vi "Generate Pulse.vi"(4 "timeout (s)":dbl=10.0 format="%0.2f", 5 "error in":errorcluster, 7 "stop (T)":bool=TRUE, 10 "device name":tag="PXIe-6341") -> (14 "task out":refnum<k21>, 19 "error out":errorcluster)   [LabVIEW 2021]
doc: "Creates, edits, and runs tasks using NI-DAQmx. Refer to the NI-DAQmx Readme for a complete listing of devices NI-DAQmx supports.\n\nWhen you place this Express VI on the block diagram, the DAQ Assistant launches to create a new task. After you create a task, you can double-click the DAQ Assistant Express VI to edit that task. For continuous measurement or generation, place a while loop around the DAQ Assistant Express VI."
uses:
  <vilib>/DAQmx/create/channels.llb/DAQmx Create Channel (CO-Pulse Generation-Time).vi
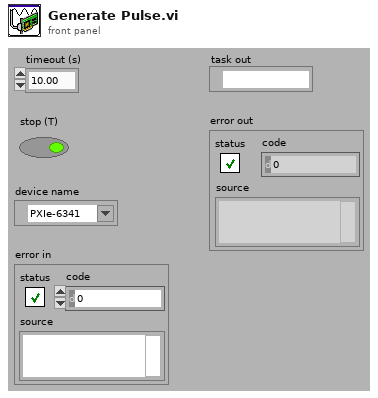
[diagram p1: front panel]
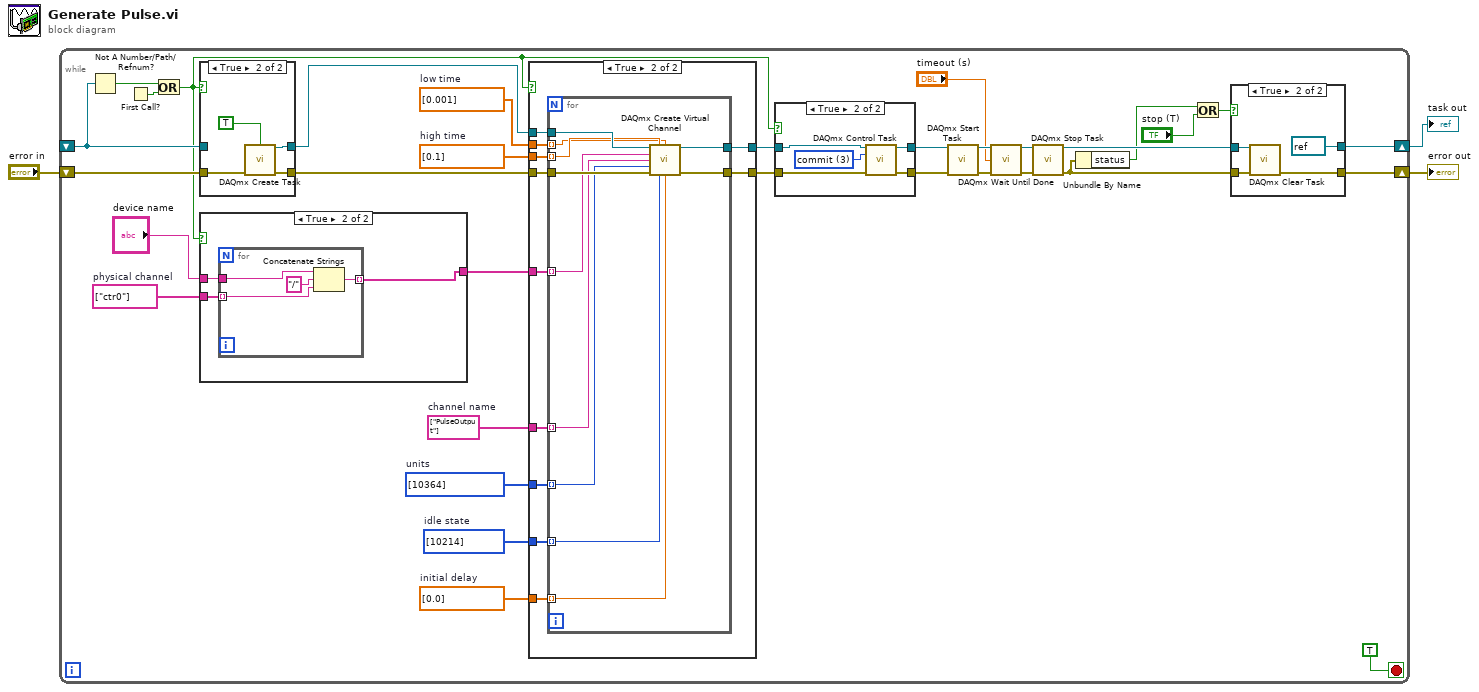
[diagram p0: block diagram]
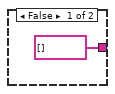
[diagram p5: hidden frame]
diagram:
  n1 = while {
    shift-right: [w10] -> w1
    shift-left: _ -> [w33]
    shift-right: [w4] -> w2
    shift-left: "error in" -> [w34]
    stop <- TRUE stop-if-true
    w21 = dbl[] [0.0]  # initial delay
    w22 = i32[] [10214] items=["High"=10192, "Low"=10214]  # idle state
    w23 = i32[] [10364] items=["Seconds"=10364, "From Custom Scale"=10065]  # units
    w24 = string[] ["PulseOutput"]  # channel name
    w26 = dbl[] [0.1]  # high time
    w27 = dbl[] [0.001]  # low time
    w30 = string[] ["ctr0"]  # physical channel
    n2 = Not A Number/Path/Refnum?(number/path/refnum=w33) -> (NaN/Path/Refnum?=w32:bool)
    n3 = First Call?() -> (First Call?: T/F=w35:bool)
    n4 = Or(x=w32, y=w35) -> (x .or. y?=w20:bool)
    n5 = case shown="True" w20 {
      tunnel: [w83 w87] -> w29
      tunnel: w33 -> [w83 _]
      tunnel: [w82 w86] -> w28
      tunnel: w34 -> [w82 w84]
      frame False {
      }
      frame True {
        n6 = call <vilib>:"DAQmx Create Task.vi"("auto cleanup"=TRUE, "error in"=w84) -> ("task out"=w87:refnum<k21>, "error out"=w86:errorcluster)  [unwired: 12 in]
      }
    }
    n7 = case shown="True" w20 {
      tunnel: [string[] [] w77] -> w25
      tunnel: "device name" -> [_ w76]
      tunnel: w30 -> [_ w75]
      frame False {
      }
      frame True {
        n8 = for {
          tunnel: [w81] -> w77 mode=indexing
          tunnel: w76 -> [w80]
          tunnel: w75 -> [w78] mode=indexing
          n9 = Concatenate Strings(w80, "/" ("string"), w78) -> (w81:string)
        }
      }
    }
    n10 = case shown="True" w20 {
      tunnel: [w51 w62] -> w19
      tunnel: w29 -> [w51 w61]
      tunnel: [w50 w60] -> w18
      tunnel: w28 -> [w50 w59]
      tunnel: w27 -> [_ w58]
      tunnel: w26 -> [_ w57]
      tunnel: w25 -> [_ w56]
      tunnel: w24 -> [_ w55]
      tunnel: w23 -> [_ w54]
      tunnel: w22 -> [_ w53]
      tunnel: w21 -> [_ w52]
      frame False {
      }
      frame True {
        n11 = for {
          tunnel: [w73] -> w62
          tunnel: w61 -> [w72]
          tunnel: [w71] -> w60
          tunnel: w59 -> [w70]
          tunnel: w56 -> [w69] mode=indexing
          tunnel: w57 -> [w68] mode=indexing
          tunnel: w58 -> [w67] mode=indexing
          tunnel: w55 -> [w66] mode=indexing
          tunnel: w54 -> [w65] mode=indexing
          tunnel: w53 -> [w64] mode=indexing
          tunnel: w52 -> [w63] mode=indexing
          n12 = call-poly <vilib>:"DAQmx Create Virtual Channel.vi"("task in"=w72, "high time"=w68, "low time"=w67, "counter"=w69, "name to assign"=w66, "units"=w65, "error in"=w70, "idle state"=w64, "initial delay"=w63) -> ("task out"=w73:refnum<k21>, "error out"=w71:errorcluster)  [unwired: 5 in]
        }
      }
    }
    n13 = case shown="True" w20 {
      tunnel: [w44 w48] -> w13
      tunnel: w19 -> [w44 w49]
      tunnel: [w43 w46] -> w12
      tunnel: w18 -> [w43 w47]
      frame False {
      }
      frame True {
        w45 = 3 items=["verify"=2, "reserve"=4, "commit"=3, "unreserve"=5, "abort"=6] ("action")
        n14 = call <vilib>:"DAQmx Control Task.vi"("task/channels in"=w49, "action"=w45, "error in"=w47) -> ("task out"=w48:refnum<k21>, "error out"=w46:errorcluster)  [unwired: 11 in]
      }
    }
    n15 = call <vilib>:"DAQmx Start Task.vi"("task/channels in"=w13, "error in"=w12) -> ("task out"=w17:refnum<k21>, "error out"=w16:errorcluster)  [unwired: 12 in]
    n16 = call <vilib>:"DAQmx Wait Until Done.vi"("task/channels in"=w17, "timeout (sec)"="timeout (s)", "error in"=w16) -> ("task out"=w14:refnum<k21>, "error out"=w15:errorcluster)  [unwired: 11 in]
    n17 = call <vilib>:"DAQmx Stop Task.vi"("task/channels in"=w14, "error in"=w15) -> ("task out"=w11:refnum<k21>, "error out"=w8:errorcluster)  [unwired: 12 in]
    n18 = Unbundle By Name(w8) -> ("status"=w7:bool)
    n19 = Or(x=w7, y="stop (T)") -> (x .or. y?=w5:bool)
    n20 = case shown="True" w5 {
      tunnel: w11 -> [w38 w42]
      tunnel: [w38 refnum<k21> refnum ("task in")] -> w10
      tunnel: w8 -> [w37 w41]
      tunnel: [w37 w40] -> w4
      frame False {
      }
      frame True {
        n21 = call <vilib>:"DAQmx Clear Task.vi"("task in"=w42, "error in"=w41) -> ("error out"=w40:errorcluster)  [unwired: 13 in]
      }
    }
  }
  "error out" <- w2
  "task out" <- w1
